vi "dvp Vi Get Trigger Jitter Filter.vi"(10 "pTriggerJitterFilter":dbl, 11 "handle":u32) -> (2 "pTriggerJitterFilter out":dbl, 3 "function return":u32(ring))   [LabVIEW 2018, in "LabViewDVPCamera.lvlib"]
doc: "LabviewDvp2Api dvpStatus dvpViGetTriggerJitterFilter(dvpHandle handle, double *pTriggerJitterFilter);"
uses:
  LabViewDVPCamera.lvlib
  LabViewDVPCamera/LabViewDVPCamera.dll
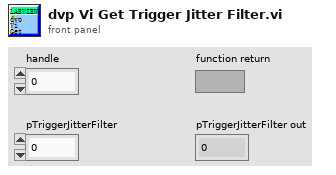
[diagram p1: front panel]
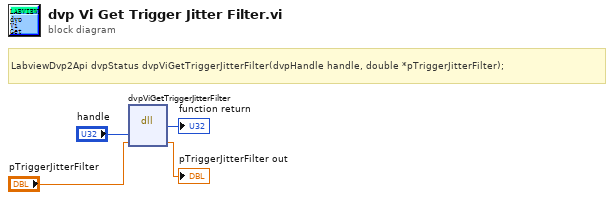
[diagram p0: block diagram]
diagram:
  # "LabviewDvp2Api dvpStatus dvpViGetTriggerJitterFilter(dvpHandle handle, double *pTriggerJitterFilter);"
  n1 = dll-call lib="C:/Program Files (x86)/DVP2 Labview cn 64/Sample/LabViewDVPCamera/LabViewDVPCamera.*" fn="dvpViGetTriggerJitterFilter"("handle"="handle", "pTriggerJitterFilter"="pTriggerJitterFilter") -> (→"function return":u32, "pTriggerJitterFilter"=→"pTriggerJitterFilter out":dbl)  [unwired: 4 in, 2 out]
